vi "Top level VI V3.vi"() -> ()   [LabVIEW 2014]
uses:
  <vilib>/Platform/TimedLoop/XDataNode/timing_clust.ctl
  <vilib>/Platform/TimedLoop/XDataNode/nitl_modes.ctl
  <vilib>/Platform/TimedLoop/XDataNode/wakeup.ctl
  <vilib>/rvi/eio/common/nirviEmuTemplateMethod_errors.vi
  <vilib>/rvi/Emulation/niFpgaSctlEmulationGetInTimedLoop.vi
  <vilib>/rvi/Emulation/niFpgaEmulationReportErrorSimple.vi
  <vilib>/rvi/Emulation/niFpgaGetClockAttributes.vi
  <vilib>/rvi/Emulation/niFpgaCriticalErrorInLSC.vi
  <vilib>/rvi/Emulation/niFpgaEmulationIsFPGAContextNoSignature.vi
  <vilib>/rvi/errors/niFpgaSetErrorForExecOnDevCompSimple.vi
  <vilib>/rvi/eio/common/nirviEmuReportErrorAndStop.vi
  <vilib>/rvi/DataTransferAndStorage/Container/Common/niFpgaContainerGetUniqueNameForEmu.vi
  <vilib>/rvi/FIFO/Fifo_Resource/nirvififoEmulationSetSize.vi
  <vilib>/rvi/FIFO/Fifo_Resource/nirviFifoEmulationQueueMgr.vi
  <instcachedir>/0/nirviFifoEmulationQueueMgr_E5CAEC123FF24DC58D834DCA3CDAA9B5.lvgen/nirviFifoEmulationQueueMgr_E5CAEC123FF24DC58D834DCA3CDAA9B5_002.vi
  <vilib>/Utility/error.llb/Clear Errors.vi
  <vilib>/rvi/FIFO/Fifo_Resource/nirvififoEmulationCreateLock.vi
  <vilib>/rvi/Emulation/niFpgaProcessEmulError.vi
  <vilib>/rvi/FIFO/Fifo_Resource/nirvififoEmulationObtainLock.vi
  <vilib>/rvi/FIFO/Fifo_Resource/nirvififoEmulationReleaseLock.vi
  <vilib>/rvi/occurrence/nirviWaitOnOccurrenceBase.vi
  <vilib>/rvi/errors/nirviReportUnexpectedCaseInternalError.vi
  <vilib>/rvi/errors/nirviReportUnexpectedCaseInternalError (U32).vi
  <vilib>/rvi/Memory/Memory_Emulation/nirvimemoryEmulation.vi
  <vilib>/rvi/Memory/Memory_Emulation/nirvimemoryFastEmulation.vi
  <vilib>/rvi/Memory/Memory_Emulation/niFpgaMemoryEmulationCacheClearOnFirstRun.vi
  <vilib>/rvi/Memory/Memory_Emulation/nirvimemoryEmulationManagerCache_MakeExclusive.vi
  <vilib>/rvi/Memory/Memory_Emulation/niFpgaMemoryEmulationValidateCache.vi
  <vilib>/rvi/Memory/Memory_Emulation/nirvimemoryEmulationManagerCache_InsertValue.vi
  <vilib>/rvi/Memory/Memory_Emulation/nirvimemoryEmulationManagerCache_ReleaseExclusive.vi
  <vilib>/rvi/Memory/Memory_Emulation/nirvimemoryEmulationManagerCache_GetValue.vi
  <vilib>/rvi/Memory/Memory_Emulation/nirvimemoryEmulationManagerCache_SetValue.vi
  <vilib>/rvi/Emulation/niFpgaSctlEmulationResourceMgr.vi
  <instcachedir>/0/nirviFifoEmulationQueueMgr_E5CAEC123FF24DC58D834DCA3CDAA9B5.lvgen/nirviFifoEmulationQueueMgr_E5CAEC123FF24DC58D834DCA3CDAA9B5_003.vi
  <vilib>/rvi/FIFO/Fifo_Resource/nirvififoEmulationDetermineInputValidOut.vi
  <vilib>/eio/EIOMethodNode/EIOMethodNode.xnode
  <vilib>/Platform/TimedLoop/XDataNode/XDataNode.xnode
  <vilib>/rvi/DataTransferAndStorage/Container/XNode/niFpgaContainer.xnode
  <vilib>/rvi/FIFO/Fifo_Resource/nirvififoEmulationRead.vi
  <vilib>/rvi/FIFO/Fifo_Resource/nirvififoEmulationWrite.vi
  <vilib>/Platform/TimedLoop/XDataNode/XDNodeRunTimeDep.lvlib
panel:
  out "Element":fxp<+/-,12,5>
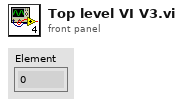
[diagram p1: front panel]
types:
  T1 = typedef "XDNodeRunTimeDep.lvlib/timing_clust.ctl" = cluster{"Expected End [f-1]":u64, "Actual End [f-1]":u64, "Finished Late? [f-1]":bool, "Expected End [i-1]":u64, "Actual End [i-1]":u64, "Finished Late? [i-1]":bool, "Expected Start [i]":u64, "Actual Start [i]":u64, "Expected Start [f]":u64, "Actual Start [f]":u64, "Source Name":string, "Structure Name":string, "Period":i64, "Deadline":i64, "Offset":i64, "Start":i64, "Priority":i32, "Timeout":i32, "Mode":T2, "Wakeup Reason":T3, "Error":errorcluster, "Source Type":string, "Secondary Source Type":string, "Global End Time":u64, "Global Start Time":u64, "Frame Duration":u64, "Iteration Duration":u64, "Assigned CPU":i32, "I/O Scan Engine Mode":u32}
  T2 = typedef "XDNodeRunTimeDep.lvlib/nitl_modes.ctl" = enum32{"No Change", "Process missed periods, maintain original phase", "Discard missed periods, maintain original phase", "Process missed periods, ignore original phase", "Discard missed periods, ignore original phase"}
  T3 = typedef "XDNodeRunTimeDep.lvlib/wakeup.ctl" = enum32{"Normal", "Aborted", "Asynchronous wakeup", "Timing source error", "Timed loop error", "Timeout"}
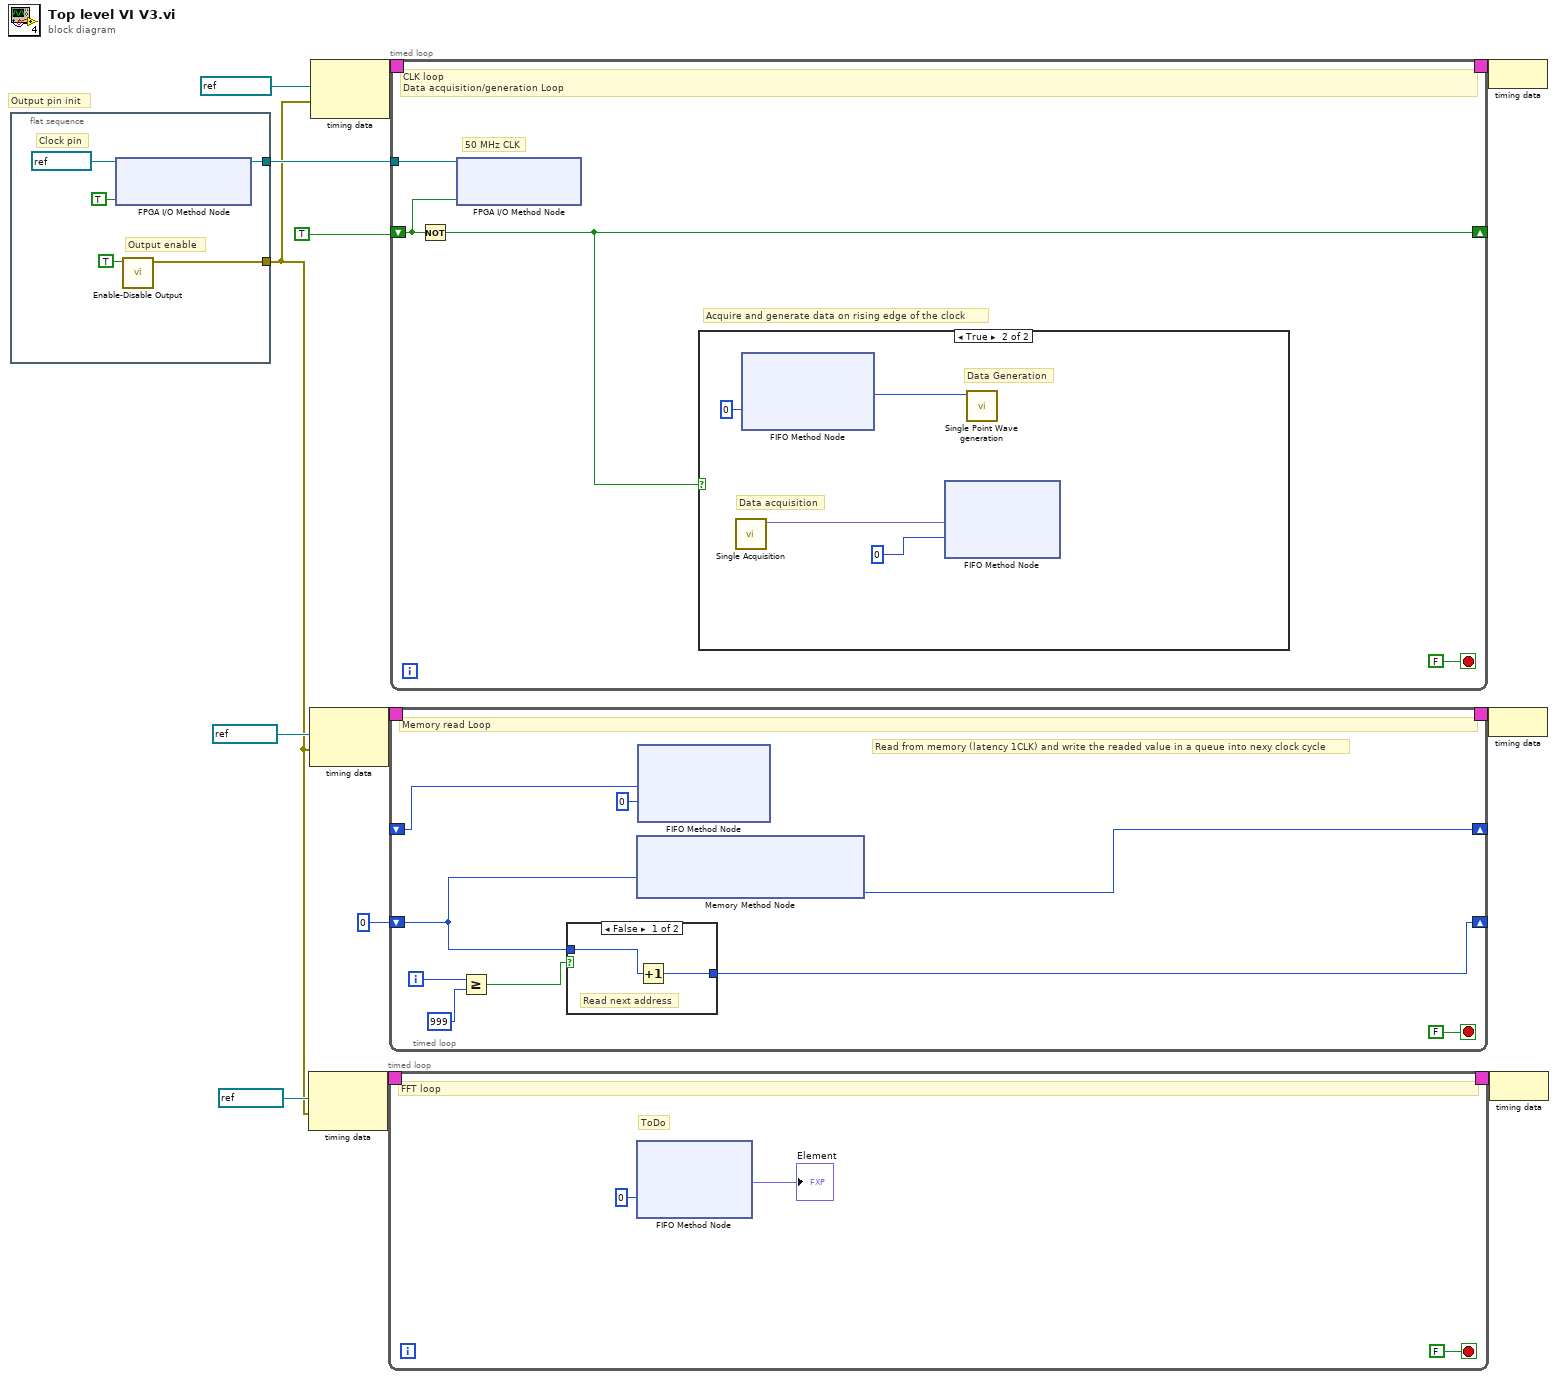
[diagram p0: block diagram]
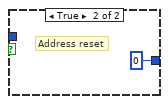
[diagram p2: hidden frame]
diagram:
  # "Output pin init"
  n1 = flat-sequence {
    tunnel: [w16] -> w9
    tunnel: [w14] -> w2
    frame #0 {
      # "Output enable"
      # "Clock pin"
      n2 = xnode "FPGA I/O Method Node"("FPGA I/O In"=refnum<k21> "DIO24", "Enable"=TRUE) -> ("FPGA I/O Out"=w16:refnum<k21>)
      n3 = call "Enable-Disable Output.vi"("Enable"=TRUE) -> ("error out"=w14:errorcluster)  [unwired: 10 in]
    }
  }
  n4 = node-c288(refnum<k21> "50MHz" ("Source Name"), w2) -> (w5:T1)
  n5 = node-c288(refnum<k21> "50MHz" ("Source Name"), w2) -> (w8:T1)
  n6 = node-c288(refnum<k21> "100MHz" ("Source Name"), w2) -> (w13:T1)
  n7 = timed-loop {
    timing: w5 -> [_]
    timing-out: [_] -> w4
    stop <- FALSE stop-if-true
    # "ToDo"
    # "FFT loop"
    n8 = xnode ("FIFO Method Node")("Timeout"=0) -> ("Element"=→"Element":fxp<+/-,12,5>)  [unwired: 1 in, 2 out]
  }
  n9 = timed-loop {
    timing: w8 -> [_]
    timing-out: [_] -> w7
    shift-right: [w32] -> _
    shift-left: _ -> [w26]
    shift-right: [w27] -> _
    shift-left: u32 0 -> [w28]
    i -> [w31]
    stop <- FALSE stop-if-true
    # "Read from memory (latency 1CLK) and write the readed value in a queue into nexy clock cycle"
    # "Memory read Loop"
    n10 = Greater Or Equal?(x=w31, y=999) -> (x >= y?=w29:bool)
    n11 = case shown="False" w29 {
      tunnel: w28 -> [w34 _]
      tunnel: [w33 u32 0] -> w27
      frame False {
        # "Read next address"
        n12 = Increment(x=w34) -> (x+1=w33:u32)
      }
      frame True {
        # "Address reset"
      }
    }
    n13 = xnode ("Memory Method Node")("Address"=w28) -> ("Data"=w32:i16)  [unwired: 1 in, 1 out]
    n14 = xnode ("FIFO Method Node")("Element"=w26, "Timeout"=0) -> ()  [unwired: 1 in, 2 out]
  }
  n15 = timed-loop {
    timing: w13 -> [_]
    timing-out: [_] -> w12
    shift-right: [w38] -> _
    shift-left: TRUE -> [w40]
    tunnel: w9 -> [w41]
    stop <- FALSE stop-if-true
    # "Acquire and generate data on rising edge of the clock"
    # "50 MHz CLK"
    # "CLK loop\nData acquisition/generation Loop"
    n16 = Not(x=w40) -> (.not. x?=w38:bool)
    n17 = xnode "FPGA I/O Method Node"("FPGA I/O In"=w41, "Data"=w40) -> ()  [unwired: 1 out]
    n18 = case shown="True" w38 {
      frame False {
      }
      frame True {
        # "Data Generation"
        # "Data acquisition"
        n19 = call "Single Acquisition.vi"() -> ("fixed-point"=w43:fxp<+/-,12,5>)  [unwired: 11 in]
        n20 = xnode ("FIFO Method Node")("Timeout"=0) -> ("Element"=w45:i16)  [unwired: 1 in, 2 out]
        n21 = xnode ("FIFO Method Node")("Element"=w43, "Timeout"=0) -> ()  [unwired: 1 in, 2 out]
        n22 = call "Single Point Wave generation.vi"("Data To Write"=w45) -> ()  [unwired: 10 in, 1 out]
      }
    }
  }
  n23 = node-c288(w12) -> ()
  n24 = node-c288(w7) -> ()
  n25 = node-c288(w4) -> ()
